vi "serial_init.vi"(0 "VISA resource name":refnum<visa-resource-name>="COM7", 1 "baud rate":u32=115200, 2 "data bits":u16=8 min=5 max=8 step=1, 3 "parity":u16(ring) items=["None", "Odd", "Even", "Mark", "Space"], 4 "stop bits":u16(ring)=10 items=["1.0"=10, "1.5"=15, "2.0"=20], 7 "flow control":u16(ring) items=["None"=0, "XON/XOFF"=1, "RTS/CTS"=2, "DTR/DSR"=4]) -> ()   [LabVIEW 2017]
doc: "The Basic Serial Read and Write example performs a Serial Port Read, a Serial Port Write, or a combination of these actions. The user selects the actions (read or write) on the front panel. If both are selected, the VI will write the data first, read data, and then close the VISA session that is opened to the port. This VI will wait until the specified number of bytes is received at the port. Only the number of bytes specified will be read.\n\nINSTRUCTIONS:\n1) Select the serial resource and configuration parameters (baud rate, data bits, parity, stop bits, flow control).\n2) Select the operations to be performed. \n3) Connect the serial port to your device. If no device is available, perform a loopback test by doing one of the following. Short pins 2 and 3 on a RS-232 cable or short pin 4 to pin 8 and pin 5 to pin 9 on a RS-485/422 cable. \n4) Run the VI to see the data read. (The \"read string\" will match the \"string to write\" if a loopback test was performed.)\n\nNote: The parameters set for the serial port must match the parameters of the connected instrument or device. In this example, the bytes to read parameter specifies the number of bytes that the serial port reads. If there were more bytes at the port than the number specified in bytes to read, those bytes would not be read. Also, if you specify to read more bytes than the number of bytes actually read, you might receive a timeout error message.\n\nOn the block diagram, the Configure Serial Port VI sets the configuration parameters. The front panel displays the controls used to configure the basic parameters, such as baud rate, data bits, and parity. Constants configure the other parameters the user probably does not need set. After the VISA Configure Serial Port VI opens the VISA session and configures the port, the VI passes the VISA resource name to other VIs that perform operations on that VISA resource. The VISA Write function sends a command to the serial device and the VISA Read function returns data based on the command. The VISA Close function then closes the reference to the serial device. It is important to close the reference; otherwise communication through with that port through protocols other than VISA might not be possible."
uses:
  <vilib>/Instr/_visa.llb/VISA Configure Serial Port (Instr).vi
panel:
  out "i":i32
  in  "Success":i32
  out "Array":string[](array[string])
  out "read string":string
  out "error out":errorcluster
  out "VISA resource name out":refnum<visa-resource-name>="COM7"
  in  "wbc":dbl=4.0
  in  "delay before read (ms)":u32=500
  # "Select the serial resource and the operations (Read, Write, or both) to be performed.  If both are selected, the VI will write the data first, read data and then close the VISA session that is opened to the port.  This VI will wait until the specified number of bytes is received at the port. Only the number of bytes specified will be read."
  # "For additional information select File >> VI Properties >> Documentation"
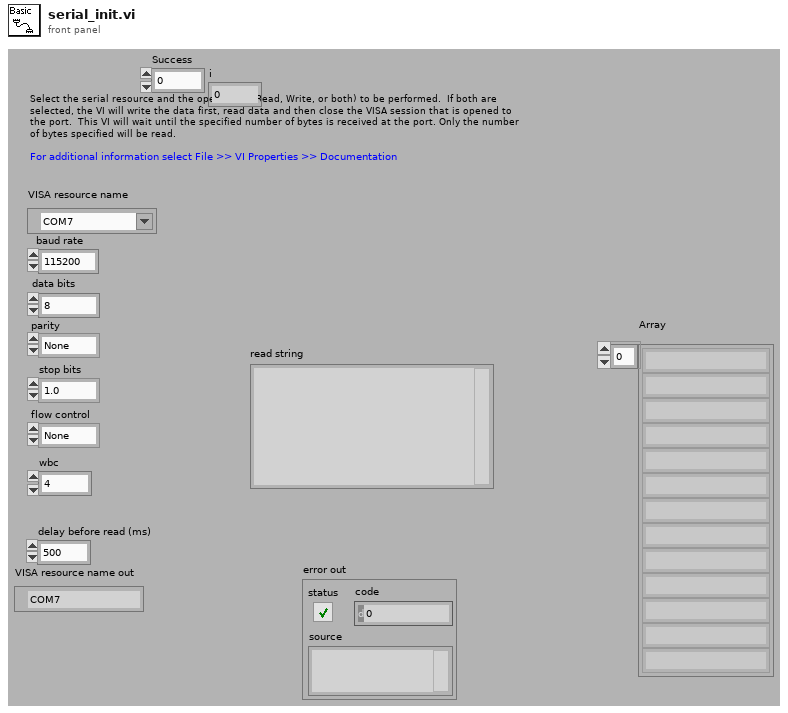
[diagram p1: front panel]
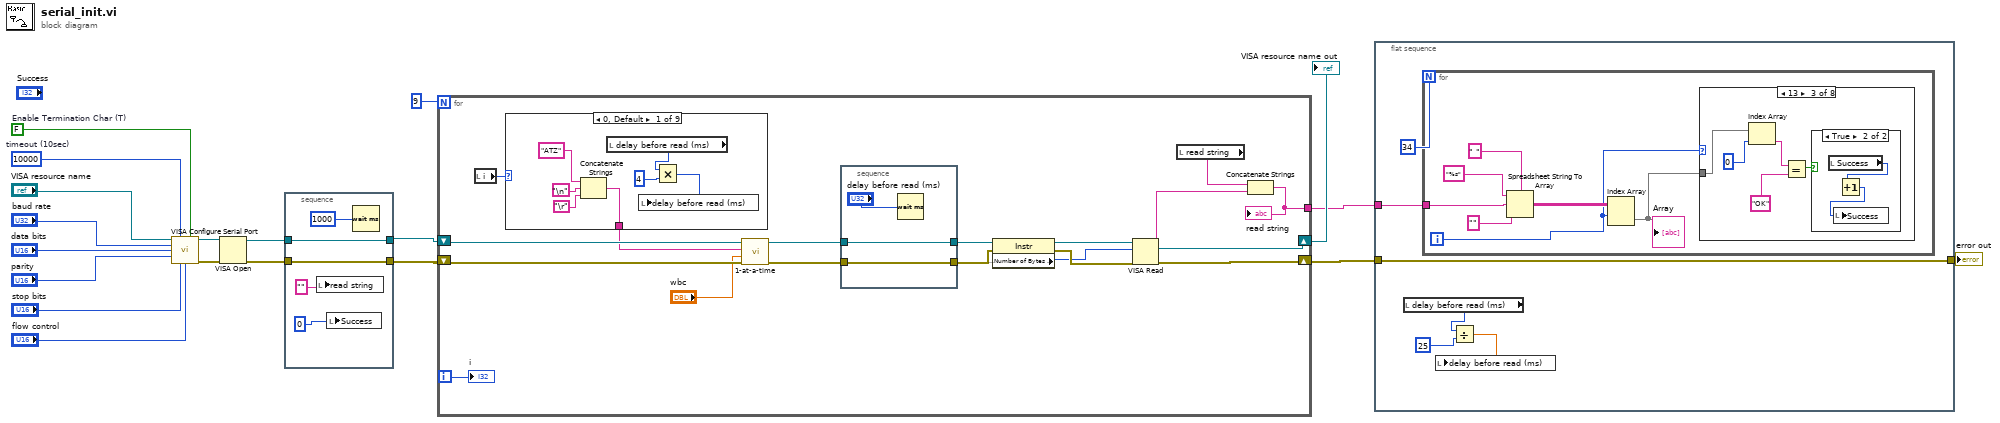
[diagram p0: block diagram]
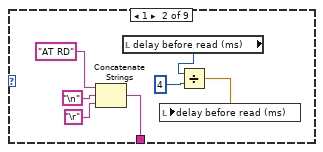
[diagram p2: hidden frame]
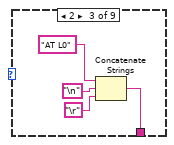
[diagram p3: hidden frame]
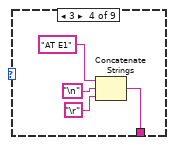
[diagram p4: hidden frame]
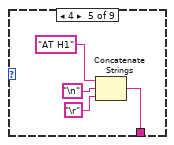
[diagram p5: hidden frame]
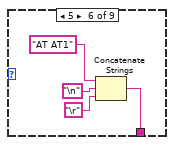
[diagram p6: hidden frame]
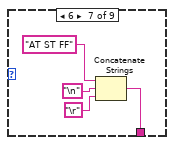
[diagram p7: hidden frame]
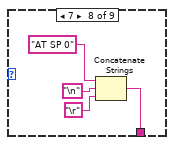
[diagram p8: hidden frame]
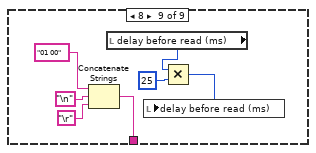
[diagram p9: hidden frame]
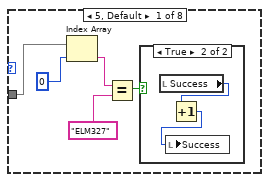
[diagram p10: hidden frame]
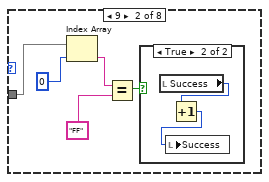
[diagram p12: hidden frame]
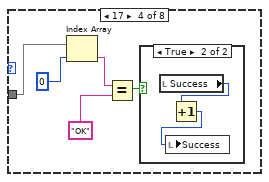
[diagram p15: hidden frame]
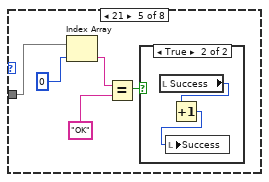
[diagram p17: hidden frame]
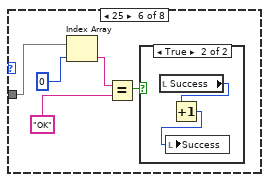
[diagram p19: hidden frame]
diagram:
  w15 = FALSE  # Enable Termination Char (T)
  w16 = u32 10000  # timeout (10sec)
  n1 = call-poly "VISA Configure Serial Port"("VISA resource name"="VISA resource name", "timeout (10sec)"=w16, "Enable Termination\nChar (T)"=w15, "baud rate (9600)"="baud rate", "data bits (8)"="data bits", "parity (0:none)"="parity", "stop bits (10: 1 bit)"="stop bits", "flow control (0:none)"="flow control") -> ("VISA resource name out"=w11:refnum<visa-resource-name>, "error out"=w10:errorcluster)  [unwired: 6 in]
  n2 = VISA Open(error in (no error)=w10, VISA resource name=w11) -> (VISA resource name=w9:refnum<visa-resource-name>, error out=w8:errorcluster)  [unwired: 3 in]
  n3 = stacked-sequence {
    tunnel: w8 -> [w24]
    tunnel: [w24] -> w6
    tunnel: w9 -> [w23]
    tunnel: [w23] -> w7
    frame #0 {
      n4 = local write "read string"("") -> ()
      n5 = local write "Success"(0) -> ()
      n6 = Wait (ms)(milliseconds to wait=u32 1000 ("delay before read (ms) 2")) -> ()  [unwired: 1 out]
    }
  }
  n7 = for {
    N: 9 -> [_]
    shift-right: [w30] -> w4
    shift-left: w6 -> [w41]
    shift-right: [w31] -> w5
    shift-left: w7 -> [w42]
    tunnel: [w29] -> w2
    i -> [w26]
    n8 = local read "i"() -> (w25:i32)
    n9 = case shown="0, Default" w25 {
      tunnel: [w49 w56 w60 w64 w68 w72 w76 w80 w87] -> w39
      frame 0, Default {
        n10 = Concatenate Strings("ATZ" ("string to write"), "\n", "\r") -> (w49:string)
        n11 = local read "delay before read (ms)"() -> (w44:u32)
        n12 = Multiply(x=w44, y=4) -> (x*y=w43:u32)
        n13 = local write "delay before read (ms)"(w43) -> ()
      }
      frame 1 {
        n14 = Concatenate Strings("AT RD" ("string to write"), "\n", "\r") -> (w56:string)
        n15 = local read "delay before read (ms)"() -> (w51:u32)
        n16 = Divide(x=w51, y=4) -> (x/y=w50:dbl)
        n17 = local write "delay before read (ms)"(w50) -> ()
      }
      frame 2 {
        n18 = Concatenate Strings("AT L0" ("string to write"), "\n", "\r") -> (w60:string)
      }
      frame 3 {
        n19 = Concatenate Strings("AT E1" ("string to write"), "\n", "\r") -> (w64:string)
      }
      frame 4 {
        n20 = Concatenate Strings("AT H1" ("string to write"), "\n", "\r") -> (w68:string)
      }
      frame 5 {
        n21 = Concatenate Strings("AT AT1" ("string to write"), "\n", "\r") -> (w72:string)
      }
      frame 6 {
        n22 = Concatenate Strings("AT ST FF" ("string to write"), "\n", "\r") -> (w76:string)
      }
      frame 7 {
        n23 = Concatenate Strings("AT SP 0" ("string to write"), "\n", "\r") -> (w80:string)
      }
      frame 8 {
        n24 = Concatenate Strings("01 00" ("string to write"), "\n", "\r") -> (w87:string)
        n25 = local read "delay before read (ms)"() -> (w82:u32)
        n26 = Multiply(x=w82, y=25) -> (x*y=w81:u32)
        n27 = local write "delay before read (ms)"(w81) -> ()
      }
    }
    n28 = call "1-at-a-time.vi"("error in (no error)"=w41, "Wait Between Characters(ms)"="wbc", "write buffer"=w39, "VISA resource name"=w42) -> ("error out"=w37:errorcluster, "VISA resource name out"=w38:refnum<visa-resource-name>)  [unwired: 5 in, 1 out]
    n29 = stacked-sequence {
      tunnel: w37 -> [w90]
      tunnel: [w90] -> w32
      tunnel: w38 -> [w89]
      tunnel: [w89] -> w33
      frame #0 {
        n30 = Wait (ms)(milliseconds to wait="delay before read (ms)") -> ()  [unwired: 1 out]
      }
    }
    n31 = property class="Instr"(reference=w33, error in=w32) -> (reference out=w36:refnum<visa-resource-name>, error out=w35:errorcluster, "Serial Settings:Number of Bytes at Serial Port"=w34:u32)
    n32 = VISA Read(VISA resource name=w36, byte count=w34, error in (no error)=w35) -> (VISA resource name out=w31:refnum<visa-resource-name>, read buffer=w27:string, error out=w30:errorcluster)  [unwired: 1 out]
    n33 = local read "read string"() -> (w28:string)
    n34 = Concatenate Strings(w28, w27) -> (w29:string)
    "read string" <- w29
    "i" <- w26
  }
  "VISA resource name out" <- w5
  n35 = flat-sequence {
    tunnel: w4 -> [w96]
    tunnel: [w96] -> w3
    tunnel: w2 -> [w95]
    frame #0 {
      n36 = local read "delay before read (ms)"() -> (w92:u32)
      n37 = for {
        N: 34 -> [_]
        tunnel: w95 -> [w99]
        i -> [w98]
        n38 = Spreadsheet String To Array(delimiter (Tab)=" ", format string="%s" ("spreadsheet string"), spreadsheet string=w99, array type (2D Dbl)="" ("spreadsheet string")) -> (array=w103:string[][])
        n39 = Index Array(array=w103, index (row)=w98) -> (element=w97:string[])  [unwired: 1 in]
        "Array" <- w97
        n40 = case shown="13" w98 {
          tunnel: w97 -> [w108 w115 w122 w129 w136 w143 w150 w157]
          frame 5, Default {
            n41 = Index Array(array=w108, index=0) -> (element=w106:string)
            n42 = Equal?(x=w106, y="ELM327") -> (x = y?=w104:bool)
            n43 = case shown="True" w104 {
              frame False {
              }
              frame True {
                n44 = local read "Success"() -> (w110:i32)
                n45 = Increment(x=w110) -> (x+1=w109:i32)
                n46 = local write "Success"(w109) -> ()
              }
            }
          }
          frame 9 {
            n47 = Index Array(array=w115, index=0) -> (element=w113:string)
            n48 = Equal?(x=w113, y="FF") -> (x = y?=w111:bool)
            n49 = case shown="True" w111 {
              frame False {
              }
              frame True {
                n50 = local read "Success"() -> (w117:i32)
                n51 = Increment(x=w117) -> (x+1=w116:i32)
                n52 = local write "Success"(w116) -> ()
              }
            }
          }
          frame 13 {
            n53 = Index Array(array=w122, index=0) -> (element=w120:string)
            n54 = Equal?(x=w120, y="OK") -> (x = y?=w118:bool)
            n55 = case shown="True" w118 {
              frame False {
              }
              frame True {
                n56 = local read "Success"() -> (w124:i32)
                n57 = Increment(x=w124) -> (x+1=w123:i32)
                n58 = local write "Success"(w123) -> ()
              }
            }
          }
          frame 17 {
            n59 = Index Array(array=w129, index=0) -> (element=w127:string)
            n60 = Equal?(x=w127, y="OK") -> (x = y?=w125:bool)
            n61 = case shown="True" w125 {
              frame False {
              }
              frame True {
                n62 = local read "Success"() -> (w131:i32)
                n63 = Increment(x=w131) -> (x+1=w130:i32)
                n64 = local write "Success"(w130) -> ()
              }
            }
          }
          frame 21 {
            n65 = Index Array(array=w136, index=0) -> (element=w134:string)
            n66 = Equal?(x=w134, y="OK") -> (x = y?=w132:bool)
            n67 = case shown="True" w132 {
              frame False {
              }
              frame True {
                n68 = local read "Success"() -> (w138:i32)
                n69 = Increment(x=w138) -> (x+1=w137:i32)
                n70 = local write "Success"(w137) -> ()
              }
            }
          }
          frame 25 {
            n71 = Index Array(array=w143, index=0) -> (element=w141:string)
            n72 = Equal?(x=w141, y="OK") -> (x = y?=w139:bool)
            n73 = case shown="True" w139 {
              frame False {
              }
              frame True {
                n74 = local read "Success"() -> (w145:i32)
                n75 = Increment(x=w145) -> (x+1=w144:i32)
                n76 = local write "Success"(w144) -> ()
              }
            }
          }
          frame 33 {
            n77 = Index Array(array=w150, index=0) -> (element=w148:string)
            n78 = Equal?(x=w148, y="SEARCHING...") -> (x = y?=w146:bool)
            n79 = case shown="True" w146 {
              frame False {
              }
              frame True {
                n80 = local read "Success"() -> (w152:i32)
                n81 = Increment(x=w152) -> (x+1=w151:i32)
                n82 = local write "Success"(w151) -> ()
              }
            }
          }
          frame 34 {
            n83 = Index Array(array=w157, index=0) -> (element=w155:string)
            n84 = Equal?(x=w155, y="86") -> (x = y?=w153:bool)
            n85 = case shown="True" w153 {
              frame False {
              }
              frame True {
                n86 = local read "Success"() -> (w159:i32)
                n87 = Increment(x=w159) -> (x+1=w158:i32)
                n88 = local write "Success"(w158) -> ()
              }
            }
          }
        }
      }
      n89 = Divide(x=w92, y=25) -> (x/y=w91:dbl)
      n90 = local write "delay before read (ms)"(w91) -> ()
    }
  }
  "error out" <- w3
